vi "roboRIO Update State.vi"(8 "error in (no error)":errorcluster, 9 "Display State In":T1, 10 "Facade Ref":refnum<vi>, 11 "Connector Ref":refnum<vi>) -> (0 "error out":errorcluster)   [LabVIEW 2021]
doc: "This VI updates Pin display in xctrl."
uses:
  <vilib>/myRIO/Common/Instrument Driver Framework/Utilities/xctls/utilities/typedefs/roboRIO Bank Display State.ctl
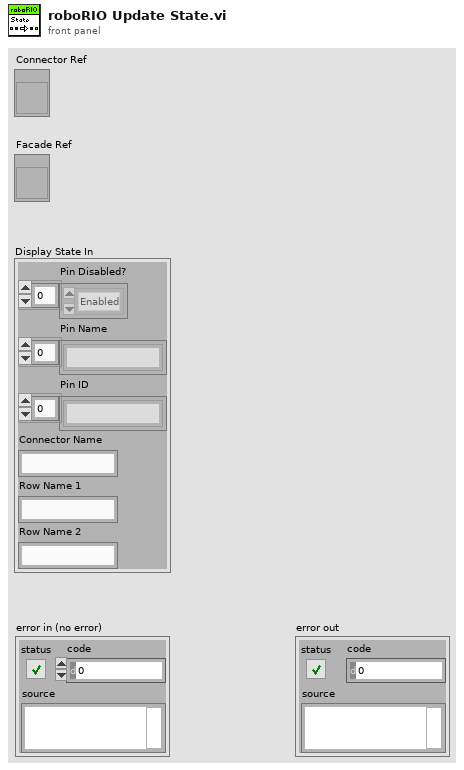
[diagram p1: front panel]
types:
  T1 = typedef "roboRIO Bank Display State.ctl" = cluster{"Pin Disabled?":enum8{"Enabled", "Disabled", "Disabled and Grayed Out"}[], "Pin Name":string[], "Pin ID":string[], "Connector Name":string, "Row Name 1":string, "Row Name 2":string}
  T2 = enum8{"Enabled", "Disabled", "Disabled and Grayed Out"}
  T3 = enum8{"Enabled", "Disabled", "Disabled and Grayed Out"}[]
  T4 = typedef "LVFontTypeDef.ctl" = cluster{"Font Name":string, "Size":u16, "Bold":bool, "Italic":bool, "Underline":bool, "Strikeout":bool, "Color":u32}
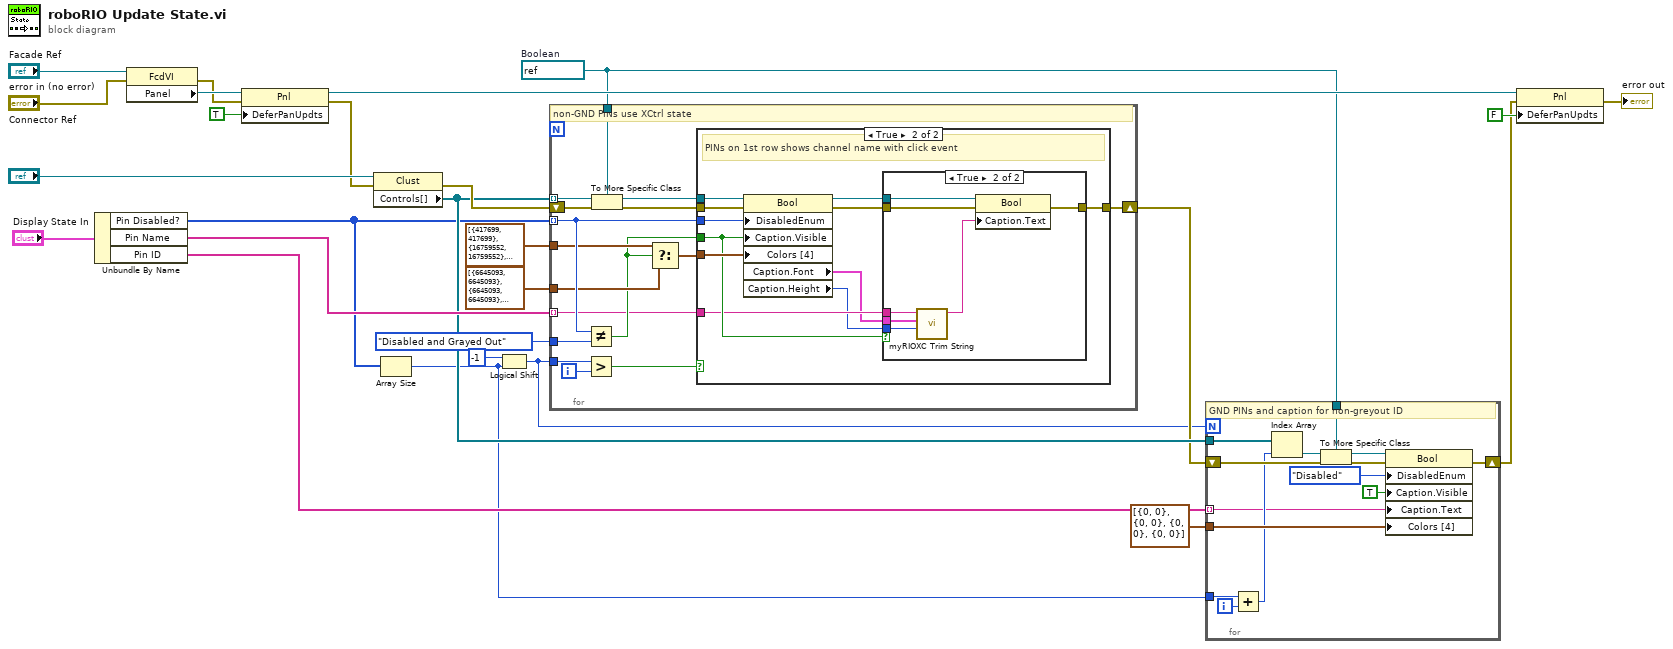
[diagram p0: block diagram]
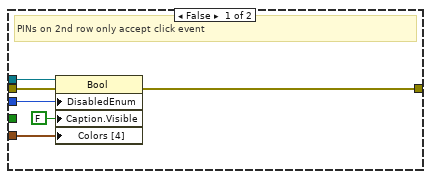
[diagram p2: hidden frame]
diagram:
  w11 = refnum<vi> refnum  # Boolean
  n1 = Unbundle By Name("Display State In") -> ("Pin Disabled?"=w8:T3, "Pin Name"=w13:string[], "Pin ID"=w9:string[])
  n2 = property class="FcdVI"(reference="Facade Ref", error in="error in (no error)") -> (error out=w17:errorcluster, "Panel"=w18:refnum<vi>)  [unwired: 1 out]
  n3 = property class="Pnl"(reference=w18, error in=w17, "DeferPanUpdts"=TRUE ("Defer Panel Updates")) -> (reference out=w21:refnum<vi>, error out=w24:errorcluster)
  n4 = property class="Clust"(reference="Connector Ref", error in=w24) -> (error out=w23:errorcluster, "Controls[]"=w10:refnum<vi>[])  [unwired: 1 out]
  n5 = Array Size(array=w8) -> (size(s)=w2:i32)
  n6 = Logical Shift(y=i16 -1, x=w2) -> (x << y=w1:i32)
  n7 = for {
    tunnel: w10 -> [w42] mode=indexing
    shift-right: [w32] -> w3
    shift-left: w23 -> [w34]
    tunnel: w8 -> [w40] mode=indexing
    tunnel: cluster{u32, u32}[] [{417699, 417699}, {16759552, 16759552}, {208721, 208721}, {8346880, 8346880}] ("Colors [4]") -> [w39]
    tunnel: cluster{u32, u32}[] [{6645093, 6645093}, {6645093, 6645093}, {6645093, 6645093}, {6645093, 6645093}] ("Colors [4]") -> [w38]
    tunnel: w13 -> [w30] mode=indexing
    tunnel: T2."Disabled and Grayed Out" ("Disabled") -> [w36]
    tunnel: w11 -> [w35]
    tunnel: w1 -> [w29]
    i -> [w28]
    # "non-GND PINs use XCtrl state"
    n8 = Not Equal?(x=w40, y=w36) -> (x != y?=w31:bool)
    n9 = Greater?(x=w29, y=w28) -> (0:w27:bool)
    n10 = To More Specific Class(target class=w35, reference=w42, error in=w34) -> (specific class reference=w41:refnum<vi>, error out=w33:errorcluster)
    n11 = Select(t=w39, s=w31, f=w38) -> (s? t:f=w37:cluster{u32, u32}[])
    n12 = case shown="True" w27 {
      tunnel: w41 -> [w48 w59]
      tunnel: w40 -> [w47 w58]
      tunnel: w37 -> [w45 w57]
      tunnel: w33 -> [w43 w56]
      tunnel: [w44 w53] -> w32
      tunnel: w31 -> [_ w52]
      tunnel: w30 -> [_ w51]
      frame False {
        # "PINs on 2nd row only accept click event"
        n13 = property class="Bool"(reference=w48, error in=w43, "DisabledEnum"=w47, "Caption.Visible"=FALSE, "Colors [4]"=w45) -> (error out=w44:errorcluster)  [unwired: 1 out]
      }
      frame True {
        # "PINs on 1st row shows channel name with click event"
        n14 = property class="Bool"(reference=w59, error in=w56, "DisabledEnum"=w58, "Caption.Visible"=w52, "Colors [4]"=w57) -> (reference out=w54:refnum<vi>, error out=w55:errorcluster, "Caption.Font"=w49:T4, "Caption.Height"=w50:u32)
        n15 = case shown="True" w52 {
          tunnel: w49 -> [_ w67]
          tunnel: w51 -> [_ w66]
          tunnel: w54 -> [_ w65]
          tunnel: w50 -> [_ w63]
          tunnel: w55 -> [w60 w62]
          tunnel: [w60 w61] -> w53
          frame False {
          }
          frame True {
            n16 = call <vilib>:"myRIOXC Trim String.vi"("Max Length"=w63, "Text Font"=w67, "Input Text"=w66) -> ("Output Text"=w64:string)  [unwired: 8 in]
            n17 = property class="Bool"(reference=w65, error in=w62, "Caption.Text"=w64) -> (error out=w61:errorcluster)  [unwired: 1 out]
          }
        }
      }
    }
  }
  n18 = for {
    N: w1 -> [_]
    shift-right: [w70] -> w6
    shift-left: w3 -> [w79]
    tunnel: w9 -> [w69] mode=indexing
    tunnel: w11 -> [w80]
    tunnel: w10 -> [w77]
    tunnel: cluster{u32, u32}[] [{0, 0}, {0, 0}, {0, 0}, {0, 0}] ("Colors [4]") -> [w74]
    tunnel: w2 -> [w72]
    i -> [w73]
    # "GND PINs and caption for non-greyout ID"
    n19 = Add(x=w72, y=w73) -> (x+y=w71:i32)
    n20 = Index Array(array=w77, index=w71) -> (element=w76:refnum<vi>)
    n21 = To More Specific Class(target class=w80, reference=w76, error in=w79) -> (specific class reference=w81:refnum<vi>, error out=w78:errorcluster)
    n22 = property class="Bool"(reference=w81, error in=w78, "DisabledEnum"=T2."Disabled" ("Disabled"), "Caption.Visible"=TRUE, "Caption.Text"=w69, "Colors [4]"=w74) -> (error out=w70:errorcluster)  [unwired: 1 out]
  }
  n23 = property class="Pnl"(reference=w21, error in=w6, "DeferPanUpdts"=FALSE ("Defer Panel Updates")) -> (error out=→"error out":errorcluster)  [unwired: 1 out]
